vi "Read Plugins State Data.vi"(8 "error in (no error)":errorcluster, 11 "Framework Status in":refnum<class "Framework Status.lvclass">) -> (0 "error out":errorcluster, 2 "plugins state data":T1[](array[typedef]) {"duration" format="%d us"}, 3 "Framework Status out":refnum<class "Framework Status.lvclass">)   [LabVIEW 2017, in "DSF Core.lvlib" / "Framework Status.lvclass"]
uses:
  Framework Status.lvclass
  Status/Status Data.ctl
  Framework Status.lvclass/Framework Status.ctl
  Status/Status Pointer.lvclass
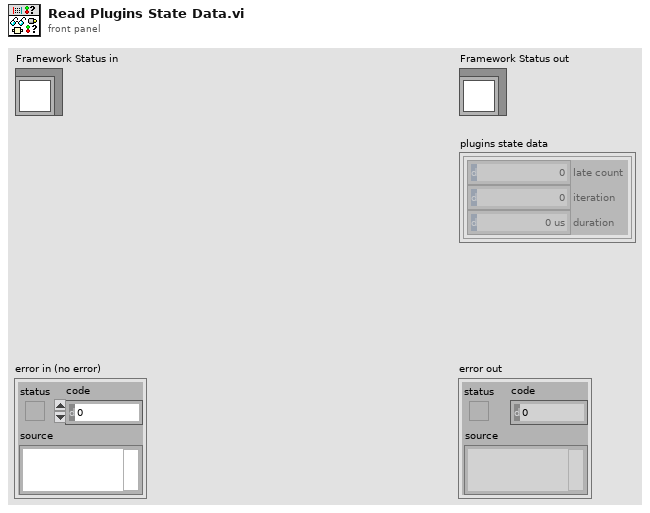
[diagram p1: front panel]
types:
  T1 = typedef "DSF Core.lvlib/Status Pointer.lvclass/Status Data.ctl" = cluster{"late count":u64, "iteration":u64, "duration":u32}
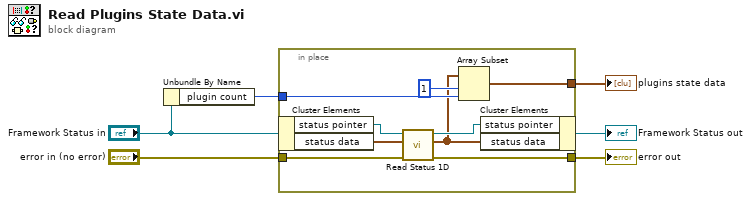
[diagram p0: block diagram]
diagram:
  n1 = Unbundle By Name("Framework Status in") -> ("plugin count"=w1:i32)
  n2 = in-place {
    in-place-border: "error in (no error)" -> [w12]
    in-place-border: [w11] -> w4
    in-place-border: [w10] -> w3
    in-place-border: w1 -> [w8]
    n3 = in-place-cluster #1("Framework Status in") -> ("status pointer"=w15:refnum<class "Status Pointer.lvclass">, "status data"=w14:T1[])
    n4 = call "Read Status 1D.vi"("error in (no error)"=w12, "statuses in"=w14, "status pointer in"=w15) -> ("error out"=w11:errorcluster, "statuses out"=w7:T1[], "status pointer out"=w13:refnum<class "Status Pointer.lvclass">)  [unwired: 6 in]
    n5 = Array Subset(array=w7, index=1, length=w8) -> (w10:T1[])
    n6 = in-place-cluster #1("status pointer"=w13, "status data"=w7) -> (→"Framework Status out":refnum<class "Framework Status.lvclass">)
  }
  "error out" <- w4
  "plugins state data" <- w3
